vi "kalman pv predict step.vi"(11 "Kalman PV state":T1) -> (3 "Kalman PV state out":T1)   [LabVIEW 2010]
uses:
  kalman pv state.ctl
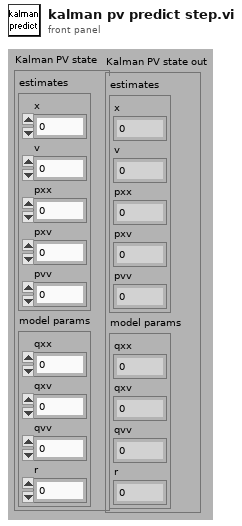
[diagram p1: front panel]
types:
  T1 = typedef "kalman pv state.ctl" = cluster{"estimates":cluster{"x":fxp<+/-,18,16>, "v":fxp<+/-,18,16>, "pxx":u16, "pxv":u16, "pvv":u16}, "model params":cluster{"qxx":u16, "qxv":u16, "qvv":u16, "r":u16}}
  T2 = cluster{"x":fxp<+/-,18,16>, "v":fxp<+/-,18,16>, "pxx":u16, "pxv":u16, "pvv":u16}
  T3 = cluster{"qxx":u16, "qxv":u16, "qvv":u16, "r":u16}
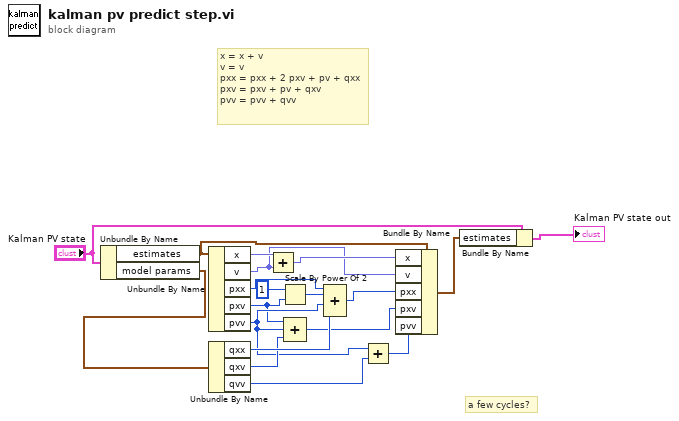
[diagram p0: block diagram]
diagram:
  # "a few cycles?"
  # "x = x + v\nv = v\npxx = pxx + 2 pxv + pv + qxx\npxv = pxv + pv + qxv\npvv = pvv + qvv"
  n1 = Unbundle By Name("Kalman PV state") -> ("estimates"=w17:T2, "model params"=w14:T3)
  n2 = Unbundle By Name(w17) -> ("x"=w19:fxp<+/-,18,16>, "v"=w15:fxp<+/-,18,16>, "pxx"=w18:u16, "pxv"=w3:u16, "pvv"=w8:u16)
  n3 = Unbundle By Name(w14) -> ("qxx"=w13:u16, "qxv"=w11:u16, "qvv"=w7:u16)
  n4 = Add(x=w19, y=w15) -> (x+y=w16:fxp<+/-,18,16>)
  n5 = Scale By Power Of 2(n=1, x=w3) -> (x*2^n=w1:u16)
  n6 = Compound Arithmetic op=ADD(w3, w8, w11) -> (w10:u16)
  n7 = Compound Arithmetic op=ADD(w18, w1, w8, w13) -> (w12:u16)
  n8 = Add(x=w8, y=w7) -> (x+y=w9:u16)
  n9 = Bundle By Name(cluster=w17, "x"=w16, "v"=w15, "pxx"=w12, "pxv"=w10, "pvv"=w9) -> (w6:T2)
  n10 = Bundle By Name(cluster="Kalman PV state", "estimates"=w6) -> (→"Kalman PV state out":T1)
